vi "Wave2D_Cal Uk_ADI W.vi"(10 "time step":i32, 11 "Wave2D Data In":T1={"PDE"={"k"=0.0, "a"=0.0, "F(t, x, y)"=[]}, "Domain"={"t"={"initial t"=0.0, "final t"=0.0, "# of t-points"=0}, "x"={"start x"=0.0, "end x"=0.0, "# of x-points"=0}, "y"={"start y"=0.0, "end y"=0.0, "# of y-points"=11}, "delta"={"delta t"=0.0, "delta x"=0.0, "delta y"=0.0}}, "BC"={"Start X"={"type"=0, "Value"=[]}, "End X"={"type"=0, "Value"=[]}, "Start Y"={"type"=0, "Value"=[]}, "End Y"={"type"=0, "Value"=[]}}, "Corner"={"Start X & Start Y"=[], "Start X & End Y"=[], "End X & Start Y"=[], "End X & End Y"=[]}, "IC"={"Value"=[], "Derivative"=[]}, "P"={"Sub Diag"=[], "Diag"=[], "Super Diag"=[], "P"=[]}, "LU of P"={"L"=[], "U"={"Diag"=[], "Super Diag"=[], "2nd Super Diag"=[]}, "Pivot"=[]}, "Q"={"Sub Diag"=[], "Diag"=[], "Super Diag"=[], "Q"=[]}, "LU of Q"={"L"=[], "U"={"Diag"=[], "Super Diag"=[], "2nd Super Diag"=[]}, "Pivot"=[]}, "State"={"U"=[], "Old U"=[], "V&W"=[], "x start index"=0, "x length"=0, "y start index"=0, "y length"=0}} {"BC"."End Y"."type" items=["Dirichlet", "Neumann"]; "BC"."Start Y"."type" items=["Dirichlet", "Neumann"]; "BC"."End X"."type" items=["Dirichlet", "Neumann"]; "BC"."Start X"."type" items=["Dirichlet", "Neumann"]}) -> (3 "Wave2D Data Out":T1={"PDE"={"k"=0.0, "a"=0.0, "F(t, x, y)"=[]}, "Domain"={"t"={"initial t"=0.0, "final t"=0.0, "# of t-points"=0}, "x"={"start x"=0.0, "end x"=0.0, "# of x-points"=0}, "y"={"start y"=0.0, "end y"=0.0, "# of y-points"=11}, "delta"={"delta t"=0.0, "delta x"=0.0, "delta y"=0.0}}, "BC"={"Start X"={"type"=0, "Value"=[]}, "End X"={"type"=0, "Value"=[]}, "Start Y"={"type"=0, "Value"=[]}, "End Y"={"type"=0, "Value"=[]}}, "Corner"={"Start X & Start Y"=[], "Start X & End Y"=[], "End X & Start Y"=[], "End X & End Y"=[]}, "IC"={"Value"=[], "Derivative"=[]}, "P"={"Sub Diag"=[], "Diag"=[], "Super Diag"=[], "P"=[]}, "LU of P"={"L"=[], "U"={"Diag"=[], "Super Diag"=[], "2nd Super Diag"=[]}, "Pivot"=[]}, "Q"={"Sub Diag"=[], "Diag"=[], "Super Diag"=[], "Q"=[]}, "LU of Q"={"L"=[], "U"={"Diag"=[], "Super Diag"=[], "2nd Super Diag"=[]}, "Pivot"=[]}, "State"={"U"=[], "Old U"=[], "V&W"=[], "x start index"=0, "x length"=0, "y start index"=0, "y length"=0}} {"BC"."End Y"."type" items=["Dirichlet", "Neumann"]; "BC"."Start Y"."type" items=["Dirichlet", "Neumann"]; "BC"."End X"."type" items=["Dirichlet", "Neumann"]; "BC"."Start X"."type" items=["Dirichlet", "Neumann"]})   [LabVIEW 2020, in "NI_PDE.lvlib"]
uses:
  <vilib>/gmath/NI_PDE.lvlib
  <vilib>/gmath/pde.llb/Wave2D/Wave2D_Data.ctl
  <vilib>/gmath/pde.llb/Common/PDE_BC Type.ctl
  <vilib>/Analysis/Matrix/Datatypes/RealMatrix.ctl
  <vilib>/Analysis/Matrix/NI_Matrix.lvlib
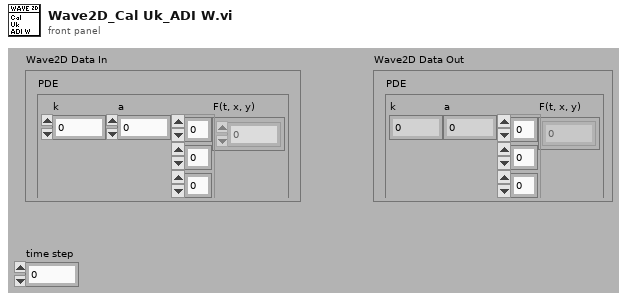
[diagram p1: front panel]
types:
  T1 = typedef "NI_PDE.lvlib/Wave2D_Data.ctl" = cluster{"PDE":cluster{"k":dbl, "a":dbl, "F(t, x, y)":dbl[][][]}, "Domain":cluster{"t":cluster{"initial t":dbl, "final t":dbl, "# of t-points":i32}, "x":cluster{"start x":dbl, "end x":dbl, "# of x-points":i32}, "y":cluster{"start y":dbl, "end y":dbl, "# of y-points":i32}, "delta":cluster{"delta t":dbl, "delta x":dbl, "delta y":dbl}}, "BC":cluster{"Start X":cluster{"type":T2, "Value":dbl[][]}, "End X":cluster{"type":T2, "Value":dbl[][]}, "Start Y":cluster{"type":T2, "Value":dbl[][]}, "End Y":cluster{"type":T2, "Value":dbl[][]}}, "Corner":cluster{"Start X & Start Y":dbl[], "Start X & End Y":dbl[], "End X & Start Y":dbl[], "End X & End Y":dbl[]}, "IC":cluster{"Value":dbl[][], "Derivative":dbl[][]}, "P":cluster{"Sub Diag":dbl[], "Diag":dbl[], "Super Diag":dbl[], "P":T3}, "LU of P":cluster{"L":dbl[], "U":cluster{"Diag":dbl[], "Super Diag":dbl[], "2nd Super Diag":dbl[]}, "Pivot":i32[]}, "Q":cluster{"Sub Diag":dbl[], "Diag":dbl[], "Super Diag":dbl[], "Q":T3}, "LU of Q":cluster{"L":dbl[], "U":cluster{"Diag":dbl[], "Super Diag":dbl[], "2nd Super Diag":dbl[]}, "Pivot":i32[]}, "State":cluster{"U":dbl[][], "Old U":dbl[][], "V&W":dbl[][], "x start index":i32, "x length":i32, "y start index":i32, "y length":i32}}
  T2 = typedef "NI_PDE.lvlib/PDE_BC Type.ctl" = i32
  T3 = typedef "NI_Matrix.lvlib/RealMatrix.ctl" = dbl[][]
  T4 = cluster{"Sub Diag":dbl[], "Diag":dbl[], "Super Diag":dbl[], "Q":T3}
  T5 = cluster{"L":dbl[], "U":cluster{"Diag":dbl[], "Super Diag":dbl[], "2nd Super Diag":dbl[]}, "Pivot":i32[]}
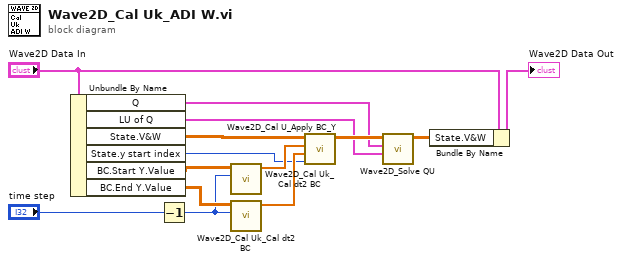
[diagram p0: block diagram]
diagram:
  n1 = Unbundle By Name("Wave2D Data In") -> ("Q"=w3:T4, "LU of Q"=w2:T5, "State.V&W"=w10:dbl[][], "State.y start index"=w7:i32, "BC.Start Y.Value"=w12:dbl[][], "BC.End Y.Value"=w11:dbl[][])
  n2 = Decrement(x="time step") -> (x-1=w1:i32)
  n3 = call <vilib>:"Wave2D_Cal Uk_Cal dt2 BC.vi"("time step"=w1, "BC Value"=w12) -> ("dt2 BC"=w9:dbl[])  [unwired: 9 out]
  n4 = call <vilib>:"Wave2D_Cal Uk_Cal dt2 BC.vi"("time step"=w1, "BC Value"=w11) -> ("dt2 BC"=w8:dbl[])  [unwired: 9 out]
  n5 = call <vilib>:"Wave2D_Cal U_Apply BC_Y.vi"("y length"=w7, "End Y Value"=w8, "Start Y Value"=w9, "U In"=w10) -> ("U Out"=w4:dbl[][])  [unwired: 7 out]
  n6 = call <vilib>:"Wave2D_Solve QU.vi"("LU of Q"=w2, "Q"=w3, "U"=w4) -> ("Q\\U"=w5:dbl[][])  [unwired: 8 out]
  n7 = Bundle By Name(cluster="Wave2D Data In", "State.V&W"=w5) -> (→"Wave2D Data Out":T1)
